vi "Main Page.vi"(8 "error in (no error)":errorcluster, 11 "Node Ptr":T1 format="%.0x") -> (0 "error out":errorcluster)   [LabVIEW 2016, in "UDP-Custom-Device System Explorer.lvlib"]
uses:
  UDP-Custom-Device System Explorer.lvlib
  <vilib>/NI Veristand/Custom Device API/Custom Device Item Ref.ctl
  Types/UDP Data Link - TypeDefs - Main Page References.ctl
  Shared/Constants.vi
  <vilib>/NI Veristand/Custom Device API/Set Item Property (Dependent Node Pointer).vi
  <vilib>/NI Veristand/Custom Device API/Set Item Property (Boolean).vi
  <vilib>/NI Veristand/Custom Device API/Set Item Property (Path).vi
  <vilib>/NI VeriStand/Custom Device API/Custom Device API.lvlib
  Shared/UDP-Custom-Device Shared.lvlib
  <vilib>/NI VeriStand/Custom Device Tools/Custom Device Utility Library/Custom Device Utility Library.lvlib
panel:
  in  "Export Path":path
  in  "Export to File on Save":bool
  in  "Export Configuration Header":cluster{"Section Name":string}={"Section Name"="UDP Export Configuration Settings"}
  in  "Select Time-Stamp Channel":bool
  out "Timestamp Channel":string
  out "Version":string
  in  "SHDocVw.IWebBrowser":refnum<k7>(container)
  in  "Network Settings Header":cluster{"Section Name":string}={"Section Name"="UDP Settings"}
  in  "General Header":cluster{"Section Name":string}={"Section Name"="UDP Custom Device Information"}
  in  "Description":string
  in  "Name":string
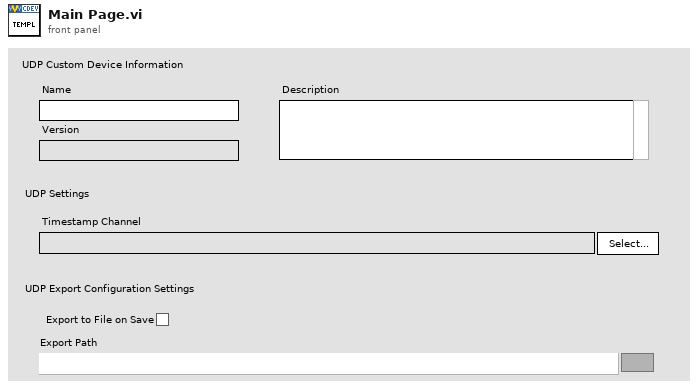
[diagram p1: front panel]
types:
  T1 = typedef "Custom Device API.lvlib/Custom Device Item Ref.ctl" = u64
  T2 = typedef "UDP-Custom-Device System Explorer.lvlib/UDP Data Link - TypeDefs - Main Page References.ctl" = cluster{"Name":refnum<vi>, "Timestamp Channel":refnum<vi>, "Export Path":refnum<vi>, "Export to File on Save":refnum<vi>}
  T3 = enum8{"Enabled", "Disabled", "Disabled and Grayed Out"}
  T4 = typedef "Custom Device API.lvlib/Custom Device Commands.ctl" = enum16{"Default", "Item renamed", "Shutdown", "Dynamic button pressed"}
  T5 = typedef "Custom Device API.lvlib/Custom Device Item Info.ctl" = cluster{"Name":string, "Is Channel":bool, "GUID":string, "Is Waveform":bool}
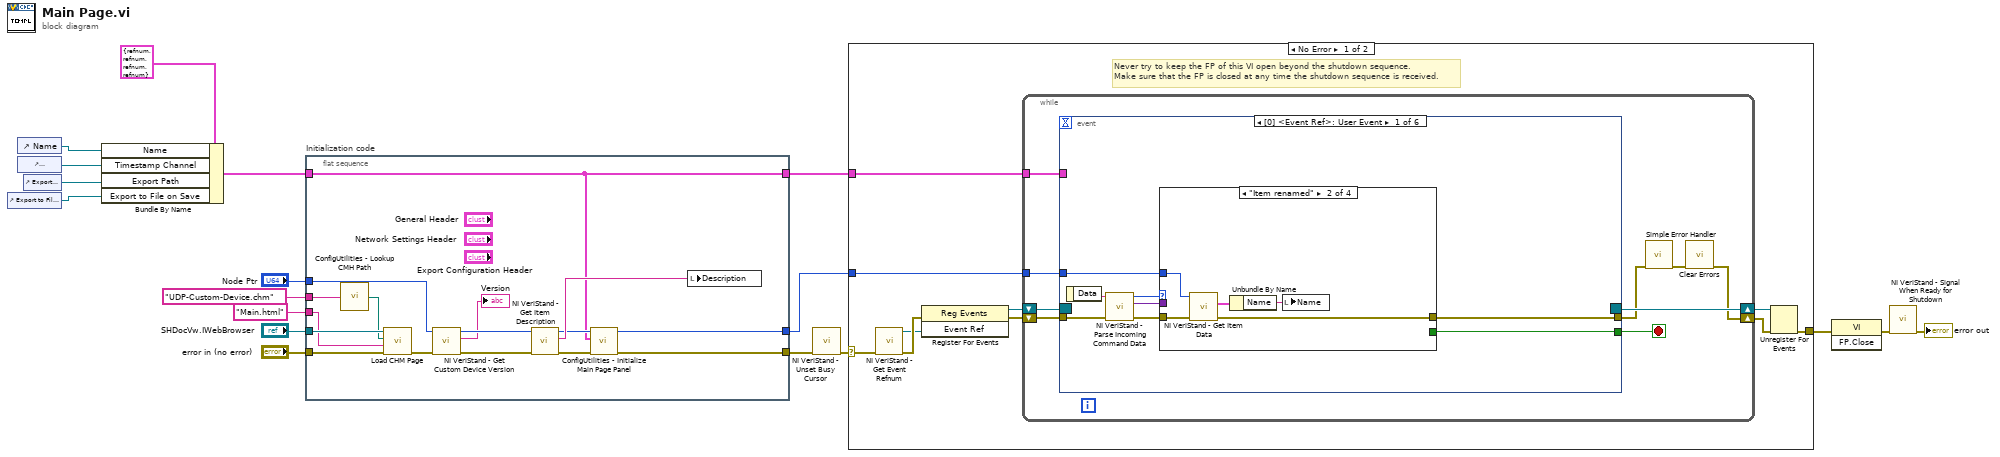
[diagram p0: block diagram]
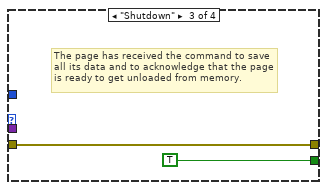
[diagram p3: hidden frame]
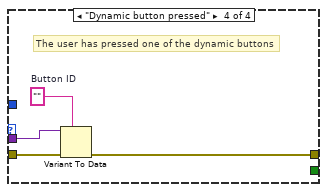
[diagram p4: hidden frame]
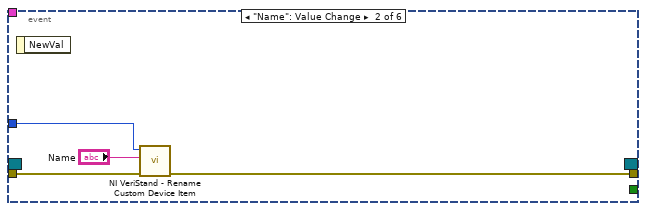
[diagram p5: hidden frame]
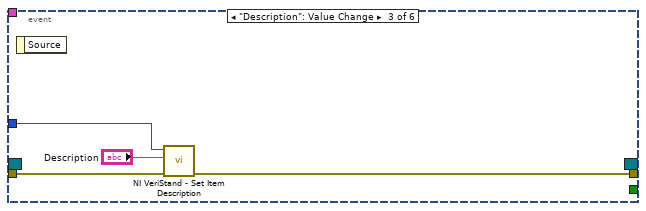
[diagram p6: hidden frame]
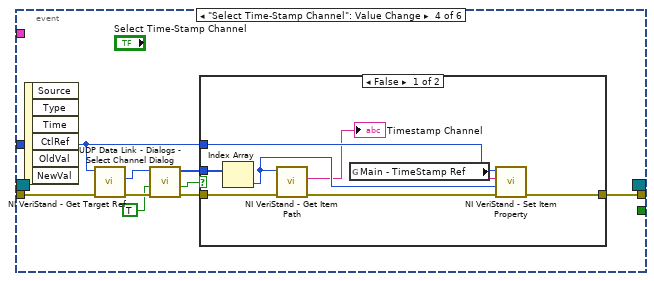
[diagram p7: hidden frame]
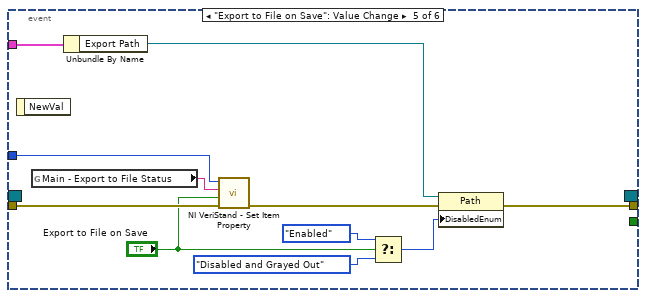
[diagram p9: hidden frame]
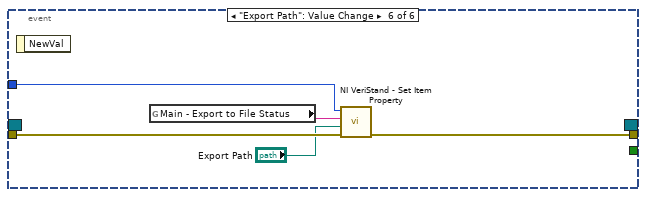
[diagram p10: hidden frame]
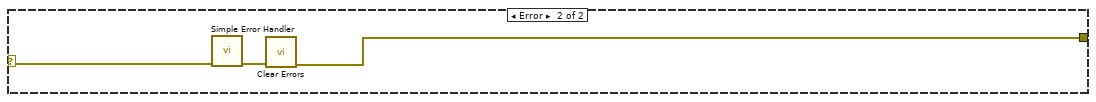
[diagram p11: hidden frame]
diagram:
  n1 = control-ref of="Export to File on Save"() -> (w4:refnum<vi>)
  n2 = control-ref of="Name"() -> (w1:refnum<vi>)
  n3 = control-ref of="Timestamp Channel"() -> (w6:refnum<vi>)
  n4 = control-ref of="Export Path"() -> (w5:refnum<vi>)
  n5 = Bundle By Name(cluster=T2 {"Name"=refnum, "Timestamp Channel"=refnum, "Export Path"=refnum, "Export to File on Save"=refnum} ("Main Page Refs"), "Name"=w1, "Timestamp Channel"=w6, "Export Path"=w5, "Export to File on Save"=w4) -> (w3:T2)
  n6 = flat-sequence "Initialization code" {
    tunnel: "error in (no error)" -> [w21]
    tunnel: "Node Ptr" -> [w34]
    tunnel: [w28] -> w14
    tunnel: [w27] -> w11
    tunnel: "SHDocVw.IWebBrowser" -> [w23]
    tunnel: "Main.html" ("HTML File") -> [w22]
    tunnel: "UDP-Custom-Device.chm" ("CD_CHM_FileName") -> [w20]
    tunnel: w3 -> [w25]
    tunnel: [w25] -> w2
    frame #0 {
      n7 = call "ConfigUtilities - Lookup CMH Path.vi"("Main CMH File"=w20) -> ("Compiled CMH Path"=w19:path)
      n8 = call <vilib>:"Load CHM Page.vi"("error in (no error)"=w21, "HTML File"=w22, "Compiled CHM Path"=w19, "Web Browser Reference"=w23) -> ("error out"=w24:errorcluster)  [unwired: 7 in]
      n9 = call <vilib>:"NI VeriStand - Get Custom Device Version.vi"("error in (no error)"=w24, "Device Ref in"=w34) -> ("error out"=w33:errorcluster, "Value"=→"Version":string, "Device Ref out"=w32:T1)  [unwired: 7 in]
      n10 = call <vilib>:"NI VeriStand - Get Item Description.vi"("error in (no error)"=w33, "Item Ref in"=w32) -> ("error out"=w29:errorcluster, "Description"=w30:string, "Item Ref out"=w26:T1)  [unwired: 7 out]
      n11 = call "ConfigUtilities - Initialize Main Page Panel.vi"("error in (no error)"=w29, "Main Page References"=w25, "Item Ref in"=w26) -> ("error out"=w28:errorcluster, "Item Ref out"=w27:T1)  [unwired: 7 in]
      n12 = local write "Description"(w30) -> ()
    }
  }
  n13 = call <vilib>:"NI VeriStand - Unset Busy Cursor.vi"("error in (no error)"=w14) -> ("error out"=w13:errorcluster)  [unwired: 10 out]
  n14 = case shown="No Error" w13 {
    selector: w13 -> [w36 w118]
    tunnel: [w41 w116] -> w18
    tunnel: w11 -> [w37 _]
    tunnel: w2 -> [w35 _]
    frame No Error {
      # "Never try to keep the FP of this VI open beyond the shutdown sequence.\nMake sure that the FP is closed at any time the shutdown sequence is received."
      n15 = call <vilib>:"NI VeriStand - Get Event Refnum.vi"("error in (no error)"=w36) -> ("error out"=w44:errorcluster, "Event Ref"=w40:refnum<user-event>)  [unwired: 9 out]
      n16 = register-events(error in=w44, w40) -> (reference out=w38:refnum<event-registration>, error out=w39:errorcluster)  [unwired: 1 in]
      n17 = while {
        tunnel: w37 -> [w49]
        shift-right: [w46] -> w42
        shift-left: w39 -> [w52]
        shift-right: [w53] -> w43
        shift-left: w38 -> [w51]
        tunnel: w35 -> [w45]
        stop <- w50 stop-if-true
        n18 = event shown="[0] <Event Ref>: User Event" {
          selector: w51 -> [_ _ _ _ _ _]
          dyn-events: [_ _ _ _ _ _] -> w53
          timeout: _ -> [_ _ _ _ _ _]
          tunnel: w52 -> [w61 w77 w80 w89 w110 w115]
          tunnel: [w57 _ _ _ _ _] -> w50
          tunnel: [w56 w76 w79 w90 w101 w114] -> w48
          tunnel: w49 -> [w55 w75 w81 w87 w109 w113]
          tunnel: w45 -> [_ _ _ _ w108 _]
          event User Event {
            n19 = event-data() -> ("Data"=w60:string)  [unwired: 1 out]
            n20 = call <vilib>:"NI VeriStand - Parse Incoming Command Data.vi"("error in (no error)"=w61, "Incoming data"=w60) -> ("error out"=w59:errorcluster, "Outgoing data"=w54:variant, "Action"=w58:T4)  [unwired: 7 out]
            n21 = case shown="\"Item renamed\"" w58 {
              tunnel: w59 -> [w62 w67 w68 w73]
              tunnel: [_ _ TRUE _] -> w57
              tunnel: [w62 w64 w68 w70] -> w56
              tunnel: w55 -> [_ w66 _ _]
              tunnel: w54 -> [_ _ _ w72]
              frame "Default", Default {
              }
              frame "Item renamed" {
                n22 = call <vilib>:"NI VeriStand - Get Item Data.vi"("error in (no error)"=w67, "Item Ref in"=w66) -> ("error out"=w64:errorcluster, "Item Info"=w65:T5)  [unwired: 8 out]
                n23 = Unbundle By Name(w65) -> ("Name"=w63:string)
                n24 = local write "Name"(w63) -> ()
              }
              frame "Shutdown" {
                # "The page has received the command to save all its data and to acknowledge that the page is ready to get unloaded from memory."
              }
              frame "Dynamic button pressed" {
                w71 = ""  # Button ID
                # "The user has pressed one of the dynamic buttons"
                n25 = Variant To Data(error in=w73, type=w71, Variant=w72) -> (error out=w70:errorcluster)  [unwired: 1 out]
              }
            }
          }
          event "Name": Value Change {
            n26 = event-data() -> ()  [unwired: 2 out]
            n27 = call <vilib>:"NI VeriStand - Rename Custom Device Item.vi"("error in (no error)"=w77, "New Name"="Name", "Item Ref in"=w75) -> ("error out"=w76:errorcluster)  [unwired: 1 in, 7 out]
          }
          event "Description": Value Change {
            n28 = event-data() -> ()  [unwired: 2 out]
            n29 = call <vilib>:"NI VeriStand - Set Item Description.vi"("error in (no error)"=w80, "Description"="Description", "Item Ref in"=w81) -> ("error out"=w79:errorcluster)  [unwired: 8 out]
          }
          event "Select Time-Stamp Channel": Value Change {
            n30 = event-data() -> ()  [unwired: 7 out]
            n31 = call <vilib>:"NI VeriStand - Get Target Ref.vi"("error in"=w89, "Item Ref in"=w87) -> ("error out"=w88:errorcluster, "Target Ref"=w86:T1)  [unwired: 6 in, 2 out]
            n32 = call "UDP Data Link - Dialogs - Select Channel Dialog.vi"("error in (no error)"=w88, "Allow Section Selection (F)"=TRUE, "Root Item Ref"=w86) -> ("error out"=w84:errorcluster, "Canceled"=w82:bool, "Selected Channel Refs"=w83:T1[])  [unwired: 6 in]
            n33 = case shown="False" w82 {
              tunnel: [w97 w99] -> w90
              tunnel: w87 -> [w96 _]
              tunnel: w84 -> [w94 w99]
              tunnel: w83 -> [w95 _]
              frame False {
                n34 = Index Array(array=w95) -> (element=w93:T1)  [unwired: 1 in]
                n35 = call <vilib>:"NI VeriStand - Get Item Path.vi"("error in (no error)"=w94, "Item Ref in"=w93) -> ("error out"=w92:errorcluster, "Path"=→"Timestamp Channel":string)  [unwired: 6 in, 2 out]
                n36 = global read "Constants.vi" "Main - TimeStamp Ref"() -> (w98:string)
                n37 = call-poly <vilib>:"NI VeriStand - Set Item Property.vi"("error in (no error)"=w92, "Dependent Node Ref"=w93, "Property Name"=w98, "Item Ref in"=w96) -> ("error out"=w97:errorcluster)  [unwired: 5 in, 2 out]
              }
              frame True {
              }
            }
          }
          event "Export to File on Save": Value Change {
            n38 = event-data() -> ()  [unwired: 2 out]
            n39 = global read "Constants.vi" "Main - Export to File Status"() -> (w100:string)
            n40 = Unbundle By Name(w108) -> ("Export Path"=w106:refnum<vi>)
            n41 = call-poly <vilib>:"NI VeriStand - Set Item Property.vi"("error in (no error)"=w110, "Value"="Export to File on Save", "Property Name"=w100, "Item Ref in"=w109) -> ("error out"=w107:errorcluster)  [unwired: 5 in, 2 out]
            n42 = Select(t=T3."Enabled" ("Disabled"), s="Export to File on Save", f=T3."Disabled and Grayed Out" ("Disabled")) -> (s? t:f=w102:T3)
            n43 = property class="Path"(reference=w106, error in=w107, "DisabledEnum"=w102) -> (error out=w101:errorcluster)  [unwired: 1 out]
          }
          event "Export Path": Value Change {
            n44 = event-data() -> ()  [unwired: 2 out]
            n45 = global read "Constants.vi" "Main - Export to File Status"() -> (w112:string)
            n46 = call-poly <vilib>:"NI VeriStand - Set Item Property.vi"("error in (no error)"=w115, "Value"="Export Path", "Property Name"=w112, "Item Ref in"=w113) -> ("error out"=w114:errorcluster)  [unwired: 5 in, 2 out]
          }
        }
        n47 = call <vilib>:"Simple Error Handler.vi"("error in (no error)"=w48) -> ("error out"=w47:errorcluster)  [unwired: 1 in, 7 out]
        n48 = call <vilib>:"Clear Errors.vi"("error in (no error)"=w47) -> ("error out"=w46:errorcluster)  [unwired: 1 in, 5 out]
      }
      n49 = Unregister For Events(event registration refnum=w43, error in=w42) -> (error out=w41:errorcluster)
    }
    frame Error {
      n50 = call <vilib>:"Simple Error Handler.vi"("error in (no error)"=w118) -> ("error out"=w117:errorcluster)  [unwired: 1 in, 7 out]
      n51 = call <vilib>:"Clear Errors.vi"("error in (no error)"=w117) -> ("error out"=w116:errorcluster)  [unwired: 1 in, 5 out]
    }
  }
  n52 = invoke class="VI" method="FP.Close"(error in=w18) -> (error out=w17:errorcluster)  [unwired: 2 in, 2 out]
  n53 = call <vilib>:"NI VeriStand - Signal When Ready for Shutdown.vi"("error in (no error)"=w17) -> ("error out"=→"error out":errorcluster)  [unwired: 10 out]
